vi "Exit.vi"(8 "error in (no error)":errorcluster) -> (0 "error out":errorcluster)   [LabVIEW 2018, in "PC UDP Reader.lvlib"]
doc: "This subVI enqueues the named action in to the communications queue along with the input data."
uses:
  PC UDP Reader.lvlib
  Private Controls/Module Data.ctl
  Private Controls/Module Action.ctl
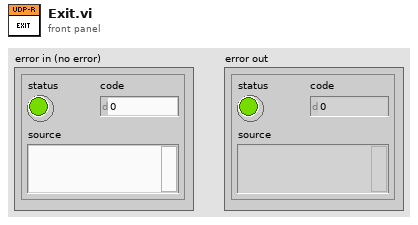
[diagram p1: front panel]
types:
  T1 = typedef "PC UDP Reader.lvlib/Module Data.ctl" = cluster{"Data":variant, "Action":T2}
  T2 = typedef "PC UDP Reader.lvlib/Module Action.ctl" = enum8{"Init", "Read", "Error", "Exit"}
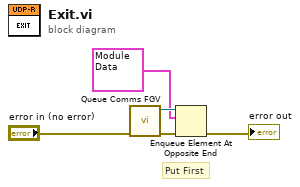
[diagram p0: block diagram]
diagram:
  # "Put First"
  n1 = call "Queue Comms FGV.vi"("error in (no error)"="error in (no error)") -> ("error out"=w5:errorcluster, "Queue out"=w4:refnum<queue>)  [unwired: 9 in]
  n2 = Enqueue Element At Opposite End(queue=w4, element=T1 {"Data"=variant, "Action"=enum."Exit"}, error in (no error)=w5) -> (error out=→"error out":errorcluster)  [unwired: 1 in, 2 out]
